vi "autostage-buildcoordinates.vi"(1 "inclusive end":bool=TRUE, 2 "Cluster":T1={"cycle-x-mod"=150, "cycle-x-range-min"=0.0, "cycle-x-range-max"=300.0, "cycle-x-step"=4.0, "cycle-y-mod"=1, "cycle-y-range-min"=0.0, "cycle-y-range-max"=300.0, "cycle-y-step"=2.0, "cycle-z-mod"=1, "cycle-z-range-min"=0.0, "cycle-z-range-max"=300.0, "cycle-z-step"=0.0}) -> (0 "coordinates":dbl[][](array[numeric]))   [LabVIEW 2017]
panel:
  out "element":dbl
  out "size(s)":i32
  out "z-values":dbl[](array[numeric])
  out "y-values":dbl[](array[numeric])
  out "x-values":dbl[](array[numeric])
  out "cycle-num":i32
  # "step\n[µm]"
  # "cycle mod"
  # "range\n[µm]"
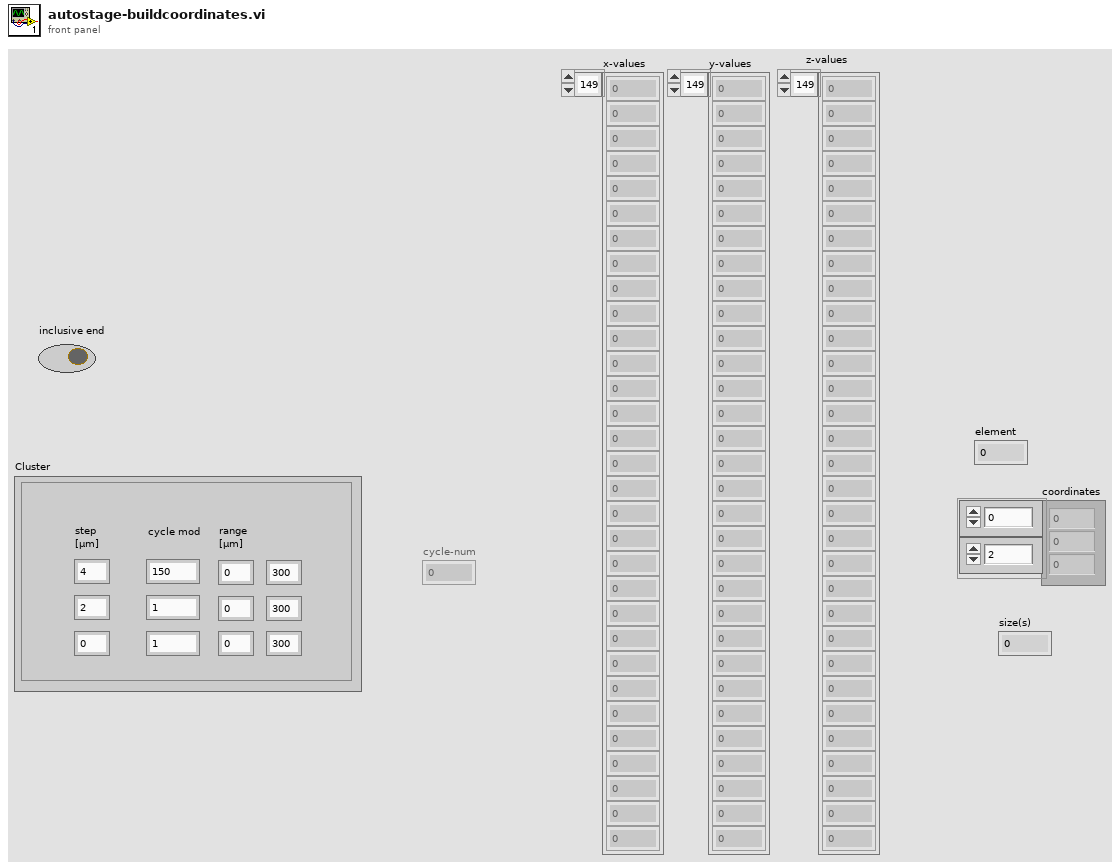
[diagram p1: front panel]
types:
  T1 = cluster{"cycle-x-mod":i32, "cycle-x-range-min":dbl, "cycle-x-range-max":dbl, "cycle-x-step":dbl, "cycle-y-mod":i32, "cycle-y-range-min":dbl, "cycle-y-range-max":dbl, "cycle-y-step":dbl, "cycle-z-mod":i32, "cycle-z-range-min":dbl, "cycle-z-range-max":dbl, "cycle-z-step":dbl}
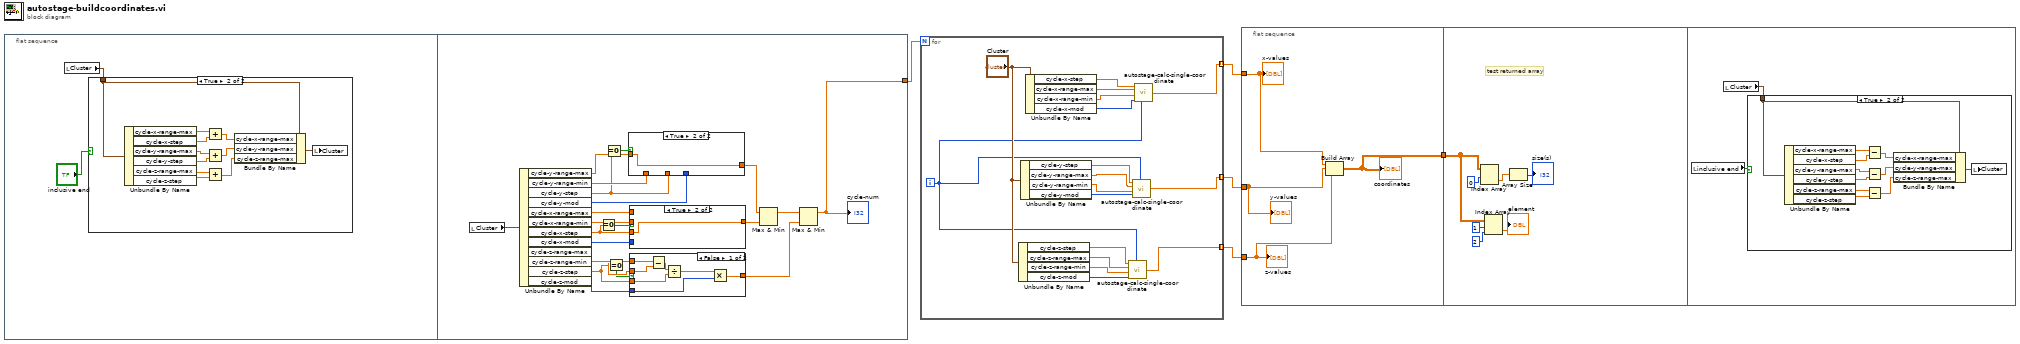
[diagram p0: block diagram]
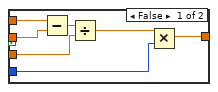
[diagram p4: hidden frame]
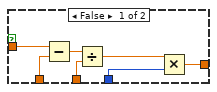
[diagram p5: hidden frame]
diagram:
  n1 = flat-sequence {
    tunnel: [w26] -> w5
    frame #0 {
      n2 = local read "Cluster"() -> (w7:T1)
      n3 = case shown="True" "inclusive end" {
        tunnel: w7 -> [_ w18]
        frame False {
        }
        frame True {
          n4 = Unbundle By Name(w18) -> ("cycle-x-range-max"=w16:dbl, "cycle-x-step"=w15:dbl, "cycle-y-range-max"=w13:dbl, "cycle-y-step"=w12:dbl, "cycle-z-range-max"=w11:dbl, "cycle-z-step"=w10:dbl)
          n5 = Add(x=w16, y=w15) -> (x+y=w14:dbl)
          n6 = Add(x=w13, y=w12) -> (x+y=w9:dbl)
          n7 = Add(x=w11, y=w10) -> (x+y=w8:dbl)
          n8 = Bundle By Name(cluster=w18, "cycle-x-range-max"=w14, "cycle-y-range-max"=w9, "cycle-z-range-max"=w8) -> (w17:T1)
          n9 = local write "Cluster"(w17) -> ()
        }
      }
    }
    frame #1 {
      n10 = local read "Cluster"() -> (w37:T1)
      n11 = Unbundle By Name(w37) -> ("cycle-y-range-max"=w36:dbl, "cycle-y-range-min"=w22:dbl, "cycle-y-step"=w19:dbl, "cycle-y-mod"=w32:i32, "cycle-x-range-max"=w35:dbl, "cycle-x-range-min"=w34:dbl, "cycle-x-step"=w20:dbl, "cycle-x-mod"=w33:i32, "cycle-z-range-max"=w31:dbl, "cycle-z-range-min"=w30:dbl, "cycle-z-step"=w24:dbl, "cycle-z-mod"=w29:i32)
      n12 = Equal To 0?(x=w20) -> (x = 0?=w21:bool)
      n13 = Equal To 0?(x=w19) -> (x = 0?=w23:bool)
      n14 = Equal To 0?(x=w24) -> (x = 0?=w25:bool)
      n15 = case shown="True" w23 {
        tunnel: [w53 w55] -> w39
        tunnel: w36 -> [w52 w55]
        tunnel: w22 -> [w51 _]
        tunnel: w19 -> [w50 _]
        tunnel: w32 -> [w49 _]
        frame False {
          n16 = Subtract(x=w52, y=w51) -> (x-y=w54:dbl)
          n17 = Divide(x=w54, y=w50) -> (x/y=w48:dbl)
          n18 = Multiply(x=w48, y=w49) -> (x*y=w53:dbl)
        }
        frame True {
        }
      }
      n19 = case shown="True" w21 {
        tunnel: [w44 w47] -> w38
        tunnel: w35 -> [w43 _]
        tunnel: w34 -> [w42 _]
        tunnel: w20 -> [w41 w47]
        tunnel: w33 -> [w40 _]
        frame False {
          n20 = Subtract(x=w43, y=w42) -> (x-y=w46:dbl)
          n21 = Divide(x=w46, y=w41) -> (x/y=w45:dbl)
          n22 = Multiply(x=w45, y=w40) -> (x*y=w44:dbl)
        }
        frame True {
        }
      }
      n23 = case shown="False" w25 {
        tunnel: w31 -> [w62 _]
        tunnel: w30 -> [w61 _]
        tunnel: w24 -> [w59 w63]
        tunnel: w29 -> [w57 _]
        tunnel: [w56 w63] -> w28
        frame False {
          n24 = Subtract(x=w62, y=w61) -> (x-y=w60:dbl)
          n25 = Divide(x=w60, y=w59) -> (x/y=w58:dbl)
          n26 = Multiply(x=w58, y=w57) -> (x*y=w56:dbl)
        }
        frame True {
        }
      }
      n27 = Max & Min(x=w39, y=w38) -> (max(x,y)=w27:dbl)  [unwired: 1 out]
      n28 = Max & Min(x=w27, y=w28) -> (max(x,y)=w26:dbl)  [unwired: 1 out]
      "cycle-num" <- w26
    }
  }
  n29 = for {
    N: w5 -> [_]
    tunnel: [w64] -> w4 mode=indexing
    tunnel: [w65] -> w3 mode=indexing
    tunnel: [w75] -> w2 mode=indexing
    i -> [w70]
    n30 = Unbundle By Name("Cluster") -> ("cycle-z-step"=w79:dbl, "cycle-z-range-max"=w78:dbl, "cycle-z-range-min"=w77:dbl, "cycle-z-mod"=w76:i32)
    n31 = Unbundle By Name("Cluster") -> ("cycle-y-step"=w69:dbl, "cycle-y-range-max"=w68:dbl, "cycle-y-range-min"=w67:dbl, "cycle-y-mod"=w66:i32)
    n32 = Unbundle By Name("Cluster") -> ("cycle-x-step"=w74:dbl, "cycle-x-range-max"=w73:dbl, "cycle-x-range-min"=w72:dbl, "cycle-x-mod"=w71:i32)
    n33 = call "autostage-calc-single-coordinate.vi"("cycle-step"=w79, "cycle-max"=w78, "cycle-min"=w77, "cycle-mod"=w76, "iterator"=w70) -> ("current-position"=w75:dbl)
    n34 = call "autostage-calc-single-coordinate.vi"("cycle-step"=w69, "cycle-max"=w68, "cycle-min"=w67, "cycle-mod"=w66, "iterator"=w70) -> ("current-position"=w65:dbl)
    n35 = call "autostage-calc-single-coordinate.vi"("cycle-step"=w74, "cycle-max"=w73, "cycle-min"=w72, "cycle-mod"=w71, "iterator"=w70) -> ("current-position"=w64:dbl)
  }
  n36 = flat-sequence {
    tunnel: w4 -> [w84]
    tunnel: w3 -> [w83]
    tunnel: w2 -> [w82]
    tunnel: [w81] -> w1
    tunnel: w1 -> [w88]
    frame #0 {
      n37 = Build Array(w84, w83, w82) -> (w81:dbl[][])
      "coordinates" <- w81
      "x-values" <- w84
      "y-values" <- w83
      "z-values" <- w82
    }
    frame #1 {
      # "test returned array"
      n38 = Index Array(array=w88, index (row)=0 ("disabled index (col)")) -> (element=w91:dbl[])  [unwired: 1 in]
      n39 = Index Array(array=w88, index (row)=1, index (col)=2 ("disabled index (col)")) -> (element=→"element":dbl)
      n40 = Array Size(array=w91) -> (size(s)=→"size(s)":i32)
    }
    frame #2 {
      n41 = local read "inclusive end"() -> (w92:bool)
      n42 = local read "Cluster"() -> (w93:T1)
      n43 = case shown="True" w92 {
        tunnel: w93 -> [_ w104]
        frame False {
        }
        frame True {
          n44 = Unbundle By Name(w104) -> ("cycle-x-range-max"=w102:dbl, "cycle-x-step"=w101:dbl, "cycle-y-range-max"=w99:dbl, "cycle-y-step"=w98:dbl, "cycle-z-range-max"=w97:dbl, "cycle-z-step"=w96:dbl)
          n45 = Subtract(x=w102, y=w101) -> (x-y=w100:dbl)
          n46 = Subtract(x=w99, y=w98) -> (x-y=w95:dbl)
          n47 = Subtract(x=w97, y=w96) -> (x-y=w94:dbl)
          n48 = Bundle By Name(cluster=w104, "cycle-x-range-max"=w100, "cycle-y-range-max"=w95, "cycle-z-range-max"=w94) -> (w103:T1)
          n49 = local write "Cluster"(w103) -> ()
        }
      }
    }
  }
